vi "Rotate to Angle Implementation.vi"(8 "Deadband (°)":dbl, 11 "Angle Setpoint":dbl) -> (0 "Finished?":bool, 3 "Numeric":dbl)   [LabVIEW 2019]
uses:
  Turret Published Globals.vi
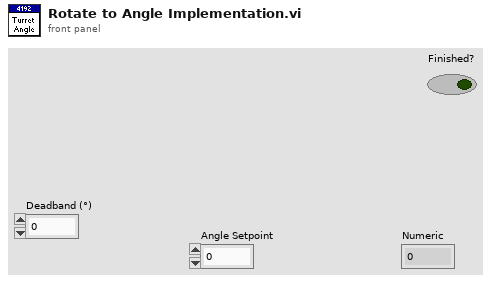
[diagram p1: front panel]
types:
  T1 = cluster{"Shooter Up To Speed?":bool, "Aligned With Target?":bool, "Hood at Angle?":bool, "Shooting?":bool, "Hood Angle":dbl, "Turret Angle":dbl, "Shooter Velocity":dbl}
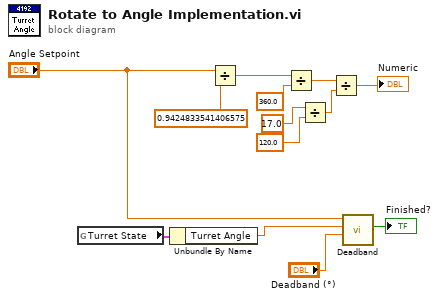
[diagram p0: block diagram]
diagram:
  n1 = global read "Turret Published Globals.vi" "Turret State"() -> (w4:T1)
  n2 = Unbundle By Name(w4) -> ("Turret Angle"=w3:dbl)
  n3 = Divide(x="Angle Setpoint", y=0.9424833541406575) -> (x/y=w12:dbl)
  n4 = Divide(x=w12, y=360.0) -> (x/y=w10:dbl)
  n5 = Divide(x=17.0, y=120.0) -> (x/y=w6:dbl)
  n6 = Divide(x=w10, y=w6) -> (x/y=→"Numeric":dbl)
  n7 = call "Deadband.vi"("Deadband"="Deadband (°)", "Value 2"=w3, "Value"="Angle Setpoint") -> ("Within Deadband?"=→"Finished?":bool)  [unwired: 8 in]
